vi "MM6.start measurement.vi"(0 "i ref in":refnum<vi>, 2 "dataFileName":string, 3 "ms timeout (10000)":i32=10000, 5 "error in (no error)":errorcluster) -> (14 "i ref out":refnum<vi>, 17 "timed out":bool, 19 "error out":errorcluster)   [LabVIEW 2014, in "MM6.lvlib"]
doc: "Starts the measurement, that has already been configured and initialized."
uses:
  MM6.lvlib
  CS_DigitalIO/PPG_ABC/PPG_ABC.PG_Running.ctl
  MM6.status.ctl
  CS_DigitalIO/PPG_ABC/PPG_ABC.lvlib
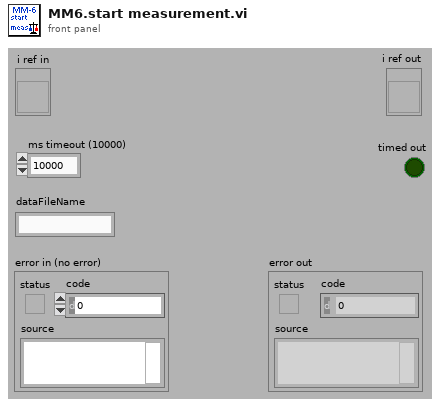
[diagram p1: front panel]
types:
  T1 = typedef "MM6.lvlib/MM6.status.ctl" = enum16{"loaded", "load_error", "config", "config_error", "init", "init_error", "data_reset", "data_reset_error", "running", "start_error", "run_error", "abort_requested", "aborted", "stop_requested", "stopped", "stop_error", "Connected", "NOTConnected"}
  T2 = typedef "PPG_ABC.lvlib/PPG_ABC.PG_Running.ctl" = i32
  T3 = typedef "MM6.lvlib/MM6.i attribute.ctl" = cluster{"ConfigData":T4, "UsedObjs":string[], "ActScanStep":i32[], "AbortRequest":bool, "StopRequest":bool, "# cycles":i32, "Connected":bool, "MMStatus":T1, "# data":i32, "DIMServices":cluster{"MM6StatusString":string, "MM6StatusID":i32, "discArchiver":string, "discArchiverID":i32, "eventBuilder":string, "eventBuilderID":i32, "GUIIDString":string, "GUIIDStringID":i32}, "dataFile":string, "ExtraDataSets":T19, "PGRunning":T2}
  T4 = typedef "LEBITDefs.lvlib/LEBITDefs.ConfigData.ctl" = cluster{"GenConfig":T5, "Configs":T7[]}
  T5 = typedef "LEBITDefs.lvlib/LEBITDefs.GenConfig.ctl" = cluster{"Mode":i32, "Logs":T6[]}
  T6 = typedef "LEBITDefs.lvlib/LEBITDefs.Log.ctl" = cluster{"Name":string, "FctName":string, "Special":string}
  T7 = typedef "LEBITDefs.lvlib/LEBITDefs.OneConfig.ctl" = cluster{"MCA":T8, "Timing":T9, "Scans":T12[], "FreqDevs":T13[], "CleanDev":T14, "NrCycles":i32, "Specials":T16[], "Delays":T17[], "DAC":T18}
  T8 = typedef "LEBITDefs.lvlib/LEBITDefs.MCA.ctl" = cluster{"Name":string, "Address":string, "NrChannels":i32, "Gate":i32, "NrPipse":i32}
  T9 = typedef "LEBITDefs.lvlib/LEBITDefs.Timing.ctl" = cluster{"TimeTables":cluster{"TimeTable":T10}[], "Memories":T11[], "ScanX":string, "ScanY":string}
  T10 = typedef "LEBITDefs.lvlib/LEBITDefs.Timetable.ctl" = dbl[]
  T11 = typedef "LEBITDefs.lvlib/LEBITDefs.Memory.ctl" = cluster{"Device":string, "ExtTrig":bool, "TT2Use":i32, "PatternTable":string[]}
  T12 = typedef "LEBITDefs.lvlib/LEBITDefs.ScanDev.ctl" = cluster{"Name":string, "FctName":string, "Values":dbl[], "NrScanVals":i32, "Special":string}
  T13 = typedef "LEBITDefs.lvlib/LEBITDefs.FreqDev.ctl" = cluster{"Name":string, "Amp":dbl, "CenterFreq":dbl, "Time":dbl}
  T14 = typedef "LEBITDefs.lvlib/LEBITDefs.CleanDev.ctl" = cluster{"Name":string, "CleanData":T15[]}
  T15 = typedef "LEBITDefs.lvlib/LEBITDefs.CleanDataType.ctl" = cluster{"Amp":dbl, "Center":dbl, "Plus":dbl, "Minus":dbl, "Time":dbl}
  T16 = typedef "LEBITDefs.lvlib/LEBITDefs.Special.ctl" = cluster{"Name":string, "FctName":string, "VerySpecial":string, "Data":dbl}
  T17 = typedef "LEBITDefs.lvlib/LEBITDefs.Delay.ctl" = cluster{"Name":string, "Delay":dbl}
  T18 = typedef "LEBITDefs.lvlib/LEBITDefs.DAC.ctl" = cluster{"Name":string, "Step1":i32, "Step2":i32}
  T19 = typedef "LEBITDefs.lvlib/LEBITDefs.ExtraData.ctl" = cluster{"Ions":cluster{"ExcitIonMass":string, "ExcitIonCharge":i32, "CleanIons":cluster{"CleanIonMass":string, "CleanIonCharge":i32}[]}, "TimingDescription":cluster{"TimeTableDescription":cluster{"Times":string[]}[], "PatternTableDescription":cluster{"Pattern":string[]}[]}, "ScanUnits":string[]}[]
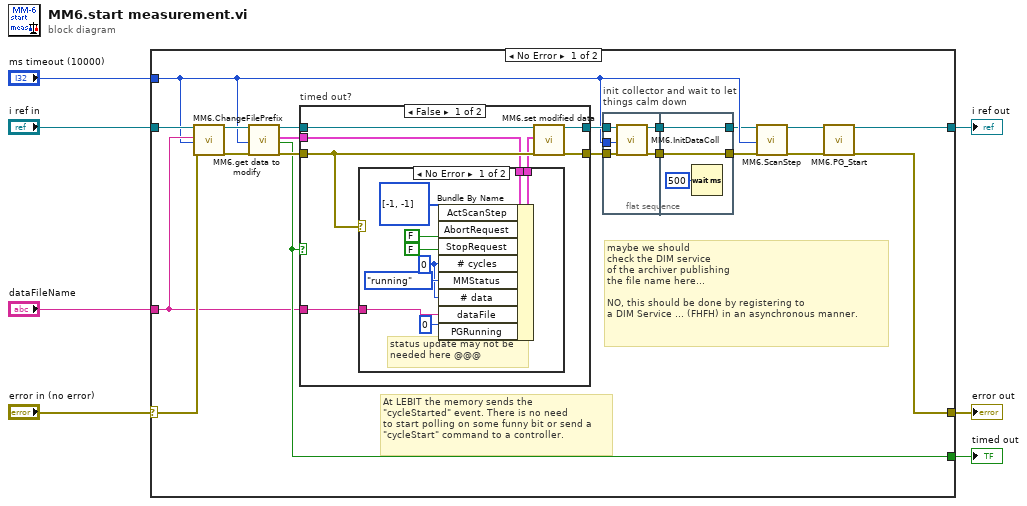
[diagram p0: block diagram]
diagram:
  n1 = case shown="No Error" "error in (no error)" {
    selector: "error in (no error)" -> [w16 w55]
    tunnel: "ms timeout (10000)" -> [w12 _]
    tunnel: [w27 w55] -> w6
    tunnel: [w26 w56] -> w5
    tunnel: [w20 _] -> w4
    tunnel: "i ref in" -> [w19 w56]
    tunnel: "dataFileName" -> [w15 _]
    frame No Error {
      # "maybe we should\ncheck the DIM service\nof the archiver publishing\nthe file name here...\n\nNO, this should be done by registering to\na DIM Service ... (FHFH) in an asynchronous manner."
      # "At LEBIT the memory sends the\n\"cycleStarted\" event. There is no need\nto start polling on some funny bit or send a\n\"cycleStart\" command to a controller."
      n2 = call "MM6.ChangeFilePrefix.vi"("i ref in"=w19, "filePrefix"=w15, "ms timeout (10000)"=w12, "error in (no error)"=w16) -> ("i ref out"=w18:refnum<vi>, "error out"=w17:errorcluster)  [unwired: 13 in, 1 out]
      n3 = call "MM6.get data to modify.vi"("i ref in"=w18, "ms timeout (10000)"=w12, "error in (no error)"=w17) -> ("i ref out"=w21:refnum<vi>, "i attribute"=w22:T3, "timed out"=w20:bool, "error out"=w23:errorcluster)  [unwired: 13 in]
      n4 = case "timed out?" shown="False" w20 {
        tunnel: w21 -> [w40 w54]
        tunnel: w22 -> [w38 _]
        tunnel: w23 -> [w39 w53]
        tunnel: [w42 w54] -> w13
        tunnel: [w41 w53] -> w14
        tunnel: w15 -> [w36 _]
        frame False {
          n5 = case shown="No Error" w39 {
            tunnel: w38 -> [w50 w52]
            tunnel: [w49 w52] -> w37
            tunnel: w36 -> [w44 _]
            frame No Error {
              w45 = 0 ("# cycles")
              # "status update may not be \nneeded here @@@"
              n6 = Bundle By Name(cluster=w50, "ActScanStep"=i32[] [-1, -1], "AbortRequest"=FALSE ("BreakRequest"), "StopRequest"=FALSE, "# cycles"=w45, "MMStatus"=MM6.status."running", "# data"=w45, "dataFile"=w44, "PGRunning"=T2 0) -> (w49:T3)
            }
            frame Error {
            }
          }
          n7 = call "MM6.set modified data.vi"("i ref in"=w40, "i attribute"=w37, "error in (no error)"=w39) -> ("i ref out"=w42:refnum<vi>, "error out"=w41:errorcluster)  [unwired: 15 in]
        }
        frame True {
        }
      }
      n8 = flat-sequence "init collector and wait to let\nthings calm down" {
        tunnel: w14 -> [w32]
        tunnel: w13 -> [w31]
        tunnel: w12 -> [w30]
        tunnel: [w29] -> w10
        tunnel: [w28] -> w8
        tunnel: [w35] -> w11
        tunnel: w10 -> [w35]
        tunnel: [w34] -> w9
        tunnel: w8 -> [w34]
        frame #0 {
          n9 = call "MM6.InitDataColl.vi"("i ref in"=w31, "ms timeout (10000)"=w30, "error in (no error)"=w32) -> ("i ref out"=w28:refnum<vi>, "error out"=w29:errorcluster)  [unwired: 14 in, 1 out]
        }
        frame #1 {
          n10 = Wait (ms)(milliseconds to wait=u32 500) -> ()  [unwired: 1 out]
        }
      }
      n11 = call "MM6.ScanStep.vi"("i ref in"=w9, "ms timeout (10000)"=w12, "error in (no error)"=w11) -> ("i ref out"=w24:refnum<vi>, "error out"=w25:errorcluster)  [unwired: 14 in, 1 out]
      n12 = call "MM6.PG_Start.vi"("i ref in"=w24, "error in (no error)"=w25) -> ("i ref out"=w26:refnum<vi>, "error out"=w27:errorcluster)  [unwired: 16 in]
    }
    frame Error {
    }
  }
  "error out" <- w6
  "i ref out" <- w5
  "timed out" <- w4
